vi "location_cal.vi"(1 "移动距离":dbl format="%#_13g", 2 "当前位置":dbl format="%#_13g", 3 "反向":bool) -> (0 "结束位置":dbl)   [LabVIEW 2018]
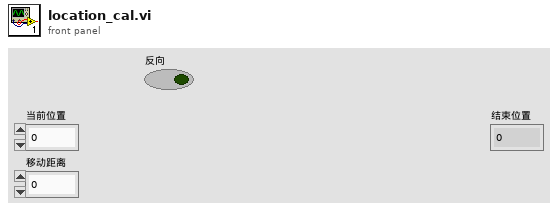
[diagram p1: front panel]
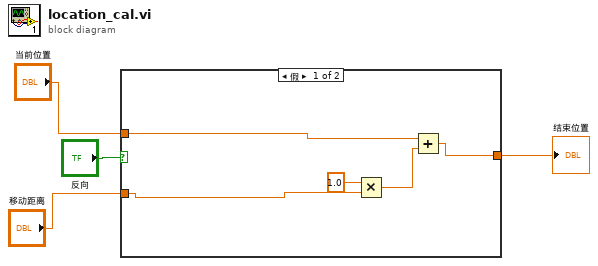
[diagram p0: block diagram]
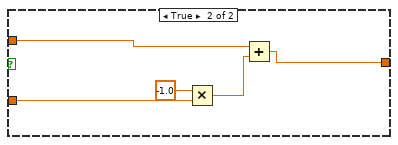
[diagram p2: hidden frame]
diagram:
  n1 = case shown="假" "反向" {
    tunnel: "当前位置" -> [w7 w14]
    tunnel: "移动距离" -> [w5 w13]
    tunnel: [w6 w10] -> w1
    frame False {
      n2 = Multiply(x=1.0, y=w5) -> (x*y=w8:dbl)
      n3 = Add(x=w7, y=w8) -> (x+y=w6:dbl)
    }
    frame True {
      n4 = Multiply(x=-1.0, y=w13) -> (x*y=w11:dbl)
      n5 = Add(x=w14, y=w11) -> (x+y=w10:dbl)
    }
  }
  "结束位置" <- w1
